vi "New Password.vi"(11 "Username":string) -> ()   [LabVIEW 2020, in "User Lib.lvlib"]
uses:
  User Lib.lvlib
  <vilib>/addons/database/Connection.llb/DB Tools Open Connec (String).vi
  <vilib>/addons/database/_DB Variant To Data/Database Variant To Data.xnode
  <vilib>/addons/database/NI_Database_API.lvlib
  Database Lib.lvlib
panel:
  out "Error out 3":errorcluster
  out "Error out 2":errorcluster
  in  "Cancel":bool
  in  "OK":bool
  in  "Old Password":string
  in  "Confirm New Password":string
  in  "New Password":string
  out "Username 2":string caption="Username"
  # "New Password"
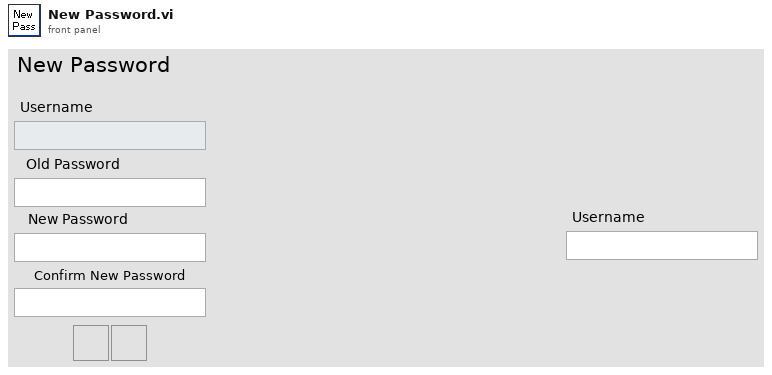
[diagram p1: front panel]
types:
  T1 = cluster{"date/time string":string, "date/time string":string, "code":i32, "date/time string":string, "source":string}
  T2 = typedef "NI_Database_API.lvlib/Conn ObjectReference.ctl" = refnum<k1>
  T3 = cluster{i32, "date/time string":string, "date/time string":string, string}
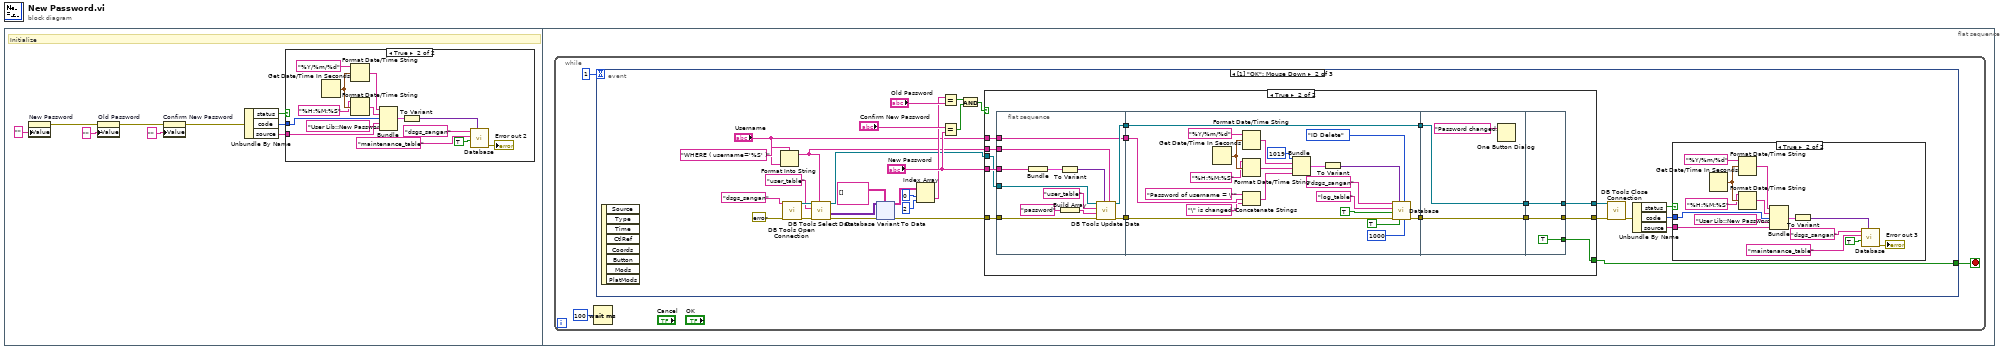
[diagram p0: block diagram]
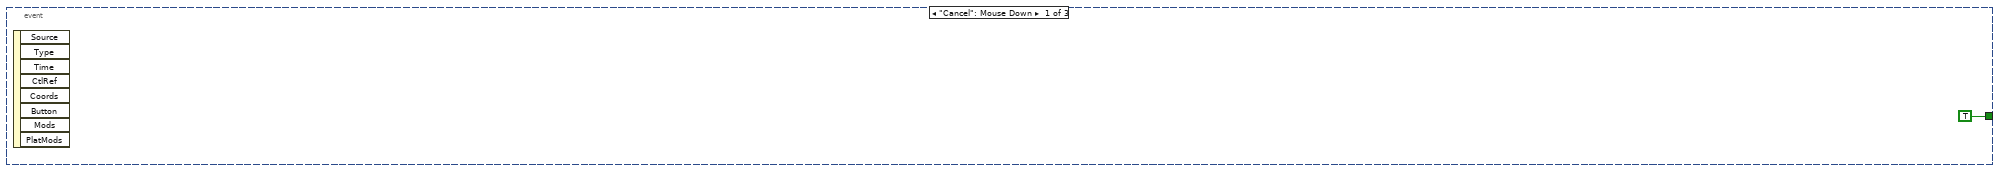
[diagram p3: hidden frame]
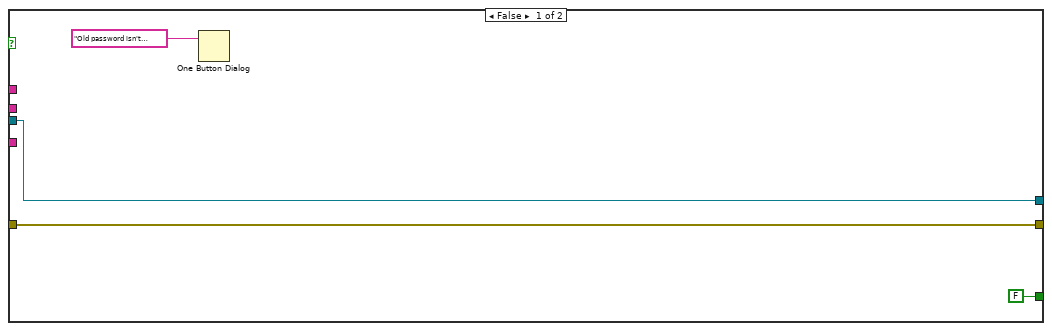
[diagram p5: hidden frame]
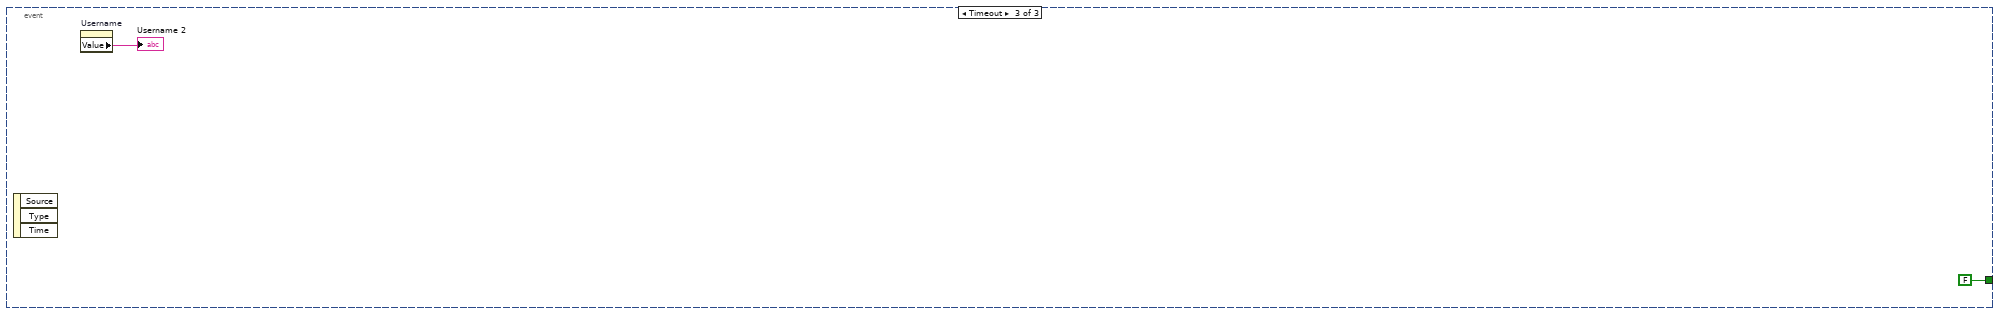
[diagram p6: hidden frame]
diagram:
  n1 = flat-sequence {
    frame #0 {
      # "Initialize"
      n2 = property on="New Password" class="Str"("Value"="" ("New Password")) -> (error out=w1:errorcluster)  [unwired: 2 in, 1 out]
      n3 = property on="Old Password" class="Str"(error in=w1, "Value"="" ("New Password")) -> (error out=w2:errorcluster)  [unwired: 1 in, 1 out]
      n4 = property on="Confirm New Password" class="Str"(error in=w2, "Value"="" ("New Password")) -> (error out=w3:errorcluster)  [unwired: 1 in, 1 out]
      n5 = Unbundle By Name(w3) -> ("status"=w5:bool, "code"=w6:i32, "source"=w4:string)
      n6 = case shown="True" w5 {
        tunnel: w6 -> [_ w18]
        tunnel: w4 -> [_ w16]
        frame False {
        }
        frame True {
          n7 = Get Date/Time In Seconds() -> (seconds since 1Jan1904=w23:timestamp)
          n8 = Format Date/Time String(time format string (%c)="%Y/%m/%d", seconds (now)=w23) -> (date/time string=w20:string)  [unwired: 1 in]
          n9 = Format Date/Time String(time format string (%c)="%H:%M:%S", seconds (now)=w23) -> (date/time string=w19:string)  [unwired: 1 in]
          n10 = Bundle("date/time string"=w20, "date/time string"=w19, "code"=w18, "date/time string"="User Lib::New Password.vi::Initialize", "source"=w16) -> (w15:T1)  [unwired: 1 in]
          n11 = To Variant(anything=w15) -> (Variant=w14:variant)
          n12 = call "Database.vi"("Data"=w14, "Auto Increment ID?"=TRUE, "Table"="maintenance_table", "Connection"="dsgs_sangan") -> ("Error out"=→"Error out 2":errorcluster)  [unwired: 7 in]
        }
      }
    }
    frame #1 {
      n13 = while {
        stop <- w25 stop-if-true
        n14 = Wait (ms)(milliseconds to wait=u32 100) -> ()  [unwired: 1 out]
        n15 = event shown="[1] \"OK\": Mouse Down" {
          selector: _ -> [_ _ _]
          dyn-events: _ -> [_ _ _]
          timeout: 1 -> [_ _ _]
          tunnel: [TRUE w34 FALSE] -> w25
          event "Cancel": Mouse Down {
            n16 = event-data() -> ()  [unwired: 1 in, 8 out]
          }
          event "OK": Mouse Down {
            n17 = event-data() -> ()  [unwired: 1 in, 8 out]
            n18 = Format Into String(format string="WHERE ( username='%S' )" ("condition"), "Username") -> (resulting string=w46:string)  [unwired: 2 in, 1 out]
            n19 = call-poly <vilib>:"DB Tools Open Connection.vi"("error in (no error)"=errorcluster {"status"=FALSE, "code"=0, "source"=""}, "connection information"="dsgs_sangan") -> ("error out"=w41:errorcluster, "connection reference"=w42:T2)  [unwired: 6 in]
            n20 = call <vilib>:"DB Tools Select Data.vi"("condition"=w46, "error in (no error)"=w41, "table"="user_table", "connection reference"=w42) -> ("error out"=w48:errorcluster, "data"=w47:variant[][], "connection reference out"=w43:T2)  [unwired: 2 in]
            n21 = xnode "Database Variant To Data"("database variant"=w47, "error in (no error)"=w48, "type"=string[][] []) -> ("data"=w50:string[][], "error out"=w49:errorcluster)
            n22 = Index Array(array=w50, index (row)=0 ("disabled index (row)"), index (col)=2 ("disabled index (col)")) -> (element=w51:string)
            n23 = Equal?(x=w51, y="Old Password") -> (x = y?=w52:bool)
            n24 = Equal?(x="Confirm New Password", y="New Password") -> (x = y?=w53:bool)
            n25 = And(x=w52, y=w53) -> (x .and. y?=w54:bool)
            n26 = case shown="True" w54 {
              tunnel: w46 -> [_ w134]
              tunnel: "New Password" -> [_ w133]
              tunnel: w49 -> [w118 w131]
              tunnel: w43 -> [w119 w132]
              tunnel: [w118 w130] -> w44
              tunnel: [w119 w129] -> w45
              tunnel: [FALSE w122] -> w34
              tunnel: "Username" -> [_ w120]
              frame False {
                n27 = One Button Dialog(message="Old password isn't correct or new password does not confirm.") -> ()  [unwired: 1 in, 1 out]
              }
              frame True {
                n28 = flat-sequence {
                  tunnel: w134 -> [w144]
                  tunnel: w133 -> [w142]
                  tunnel: w132 -> [w139]
                  tunnel: w131 -> [w138]
                  tunnel: [w137] -> w128
                  tunnel: [w136] -> w127
                  tunnel: [w135] -> w121
                  tunnel: w120 -> [w135]
                  tunnel: w128 -> [w154]
                  tunnel: w127 -> [w167]
                  tunnel: [w153] -> w126
                  tunnel: [w167] -> w125
                  tunnel: w121 -> [w151]
                  tunnel: w126 -> [w170]
                  tunnel: w125 -> [w169]
                  tunnel: [w170] -> w124
                  tunnel: [w169] -> w123
                  tunnel: [w172] -> w129
                  tunnel: [w173] -> w130
                  tunnel: w124 -> [w173]
                  tunnel: w123 -> [w172]
                  tunnel: [TRUE] -> w122
                  frame #0 {
                    n29 = Bundle("New Password"=w142) -> (w141:cluster{"New Password":string})  [unwired: 1 in]
                    n30 = To Variant(anything=w141) -> (Variant=w140:variant)
                    n31 = Build Array("password" ("table")) -> (w146:string[])
                    n32 = call <vilib>:"DB Tools Update Data.vi"("condition"=w144, "data"=w140, "error in (no error)"=w138, "columns"=w146, "table"="user_table", "connection reference"=w139) -> ("error out"=w137:errorcluster, "connection reference out"=w136:T2)  [unwired: 4 in]
                  }
                  frame #1 {
                    n33 = Get Date/Time In Seconds() -> (seconds since 1Jan1904=w162:timestamp)
                    n34 = Format Date/Time String(time format string (%c)="%Y/%m/%d", seconds (now)=w162) -> (date/time string=w163:string)  [unwired: 1 in]
                    n35 = Format Date/Time String(time format string (%c)="%H:%M:%S", seconds (now)=w162) -> (date/time string=w164:string)  [unwired: 1 in]
                    n36 = Concatenate Strings("Password of username = \"" ("string"), w151, "\" is changed." ("string")) -> (w150:string)
                    n37 = Bundle(1019, "date/time string"=w163, "date/time string"=w164, w150) -> (w165:T3)  [unwired: 1 in]
                    n38 = To Variant(anything=w165) -> (Variant=w166:variant)
                    n39 = call "Database.vi"("Maximum Row"=1000, "Enum"=enum16{"ID Delete", "Time Delete"}."ID Delete", "Delete row?"=TRUE, "Data"=w166, "Error in"=w154, "Auto Increment ID?"=TRUE, "Table"="log_table" ("table"), "Connection"="dsgs_sangan" ("table")) -> ("Error out"=w153:errorcluster)  [unwired: 3 in]
                  }
                  frame #2 {
                    n40 = One Button Dialog(message="Password changed.") -> ()  [unwired: 1 in, 1 out]
                  }
                  frame #3 {
                  }
                }
              }
            }
            n41 = call <vilib>:"DB Tools Close Connection.vi"("error in (no error)"=w44, "connection reference"=w45) -> ("error out"=w29:errorcluster)  [unwired: 5 in]
            n42 = Unbundle By Name(w29) -> ("status"=w31:bool, "code"=w32:i32, "source"=w30:string)
            n43 = case shown="True" w31 {
              tunnel: w32 -> [_ w66]
              tunnel: w30 -> [_ w64]
              frame False {
              }
              frame True {
                n44 = Get Date/Time In Seconds() -> (seconds since 1Jan1904=w71:timestamp)
                n45 = Format Date/Time String(time format string (%c)="%Y/%m/%d", seconds (now)=w71) -> (date/time string=w68:string)  [unwired: 1 in]
                n46 = Format Date/Time String(time format string (%c)="%H:%M:%S", seconds (now)=w71) -> (date/time string=w67:string)  [unwired: 1 in]
                n47 = Bundle("date/time string"=w68, "date/time string"=w67, "code"=w66, "date/time string"="User Lib::New Password.vi::\"OK\" case", "source"=w64) -> (w63:T1)  [unwired: 1 in]
                n48 = To Variant(anything=w63) -> (Variant=w62:variant)
                n49 = call "Database.vi"("Data"=w62, "Auto Increment ID?"=TRUE, "Table"="maintenance_table", "Connection"="dsgs_sangan") -> ("Error out"=→"Error out 3":errorcluster)  [unwired: 7 in]
              }
            }
          }
          event Timeout {
            n50 = event-data() -> ()  [unwired: 1 in, 3 out]
            n51 = property on="Username" class="Str"() -> ("Value"=→"Username 2":string)  [unwired: 2 in, 2 out]
          }
        }
      }
    }
  }
